vi "Gif.Header.vi"(0 "data":string, 9 "offset":i32, 11 "error in (no error)":errorcluster) -> (4 "data out":string, 6 "Signature":string, 8 "Version":string, 10 "offset out":i32, 15 "error out":errorcluster)   [LabVIEW 2011]
doc: "This vi reads the header information from the loaded file. If the file is a gif file, then the first three bytes contain \"GIF\" and the second three bytes contain the version (\"87a\", \"89a\")."
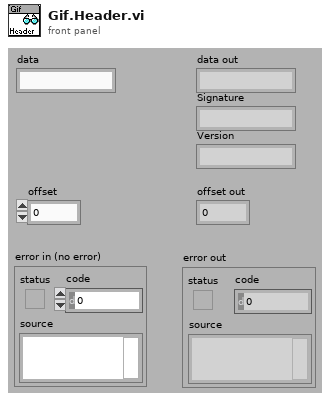
[diagram p1: front panel]
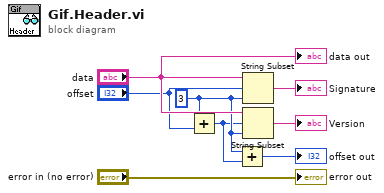
[diagram p0: block diagram]
diagram:
  w3 = 3 ("length (rest)")
  n1 = Add(x=w3, y="offset") -> (x+y=w2:i32)
  n2 = Add(x=w3, y=w2) -> (x+y=→"offset out":i32)
  n3 = String Subset(string="data", offset (0)="offset", length (rest)=w3) -> (substring=→"Signature":string)
  n4 = String Subset(string="data", offset (0)=w2, length (rest)=w3) -> (substring=→"Version":string)
  "data out" <- "data"
  "error out" <- "error in (no error)"
